vi "DetPars.vi"(1 "Immediate":bool=TRUE) -> (0 "status":i32)   [LabVIEW 2014]
uses:
  globals/DetectorGlobals.vi
panel:
  in  "FullFrame":bool caption="Boolean"
  in  "Last \nColumn":i32=4096 min=1 step=1
  in  "Last\nRow":i32=4096 min=1 step=1
  in  "Row\nBin":i32=3 min=1 max=100 step=1
  in  "Column\nBin":i32=5 min=1 max=100 step=1
  in  "First \nColumn":i32=1 min=1 step=1
  in  "First\nRow":i32=1 min=1 step=1
  in  "OK":bool caption="Boolean"
  in  "Apply":bool caption="Boolean"
  in  "Quit":bool
  in  "Close":bool caption="Boolean"
  # "Detector Region-Of-Interest"
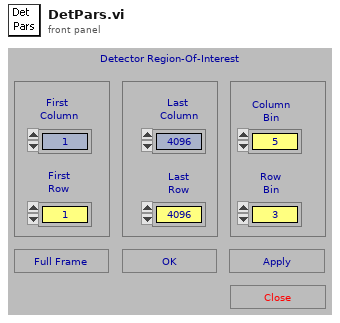
[diagram p1: front panel]
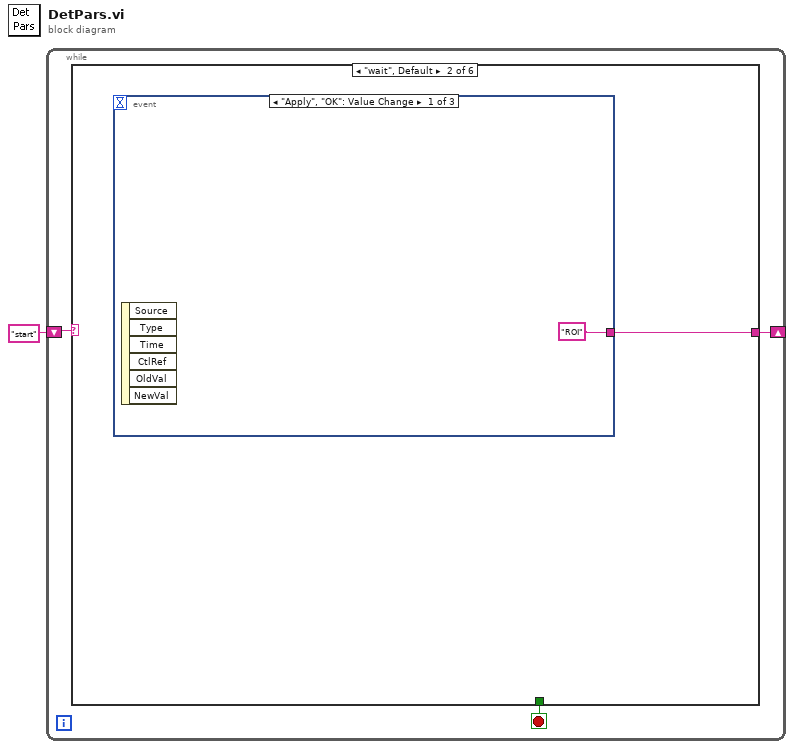
[diagram p0: block diagram]
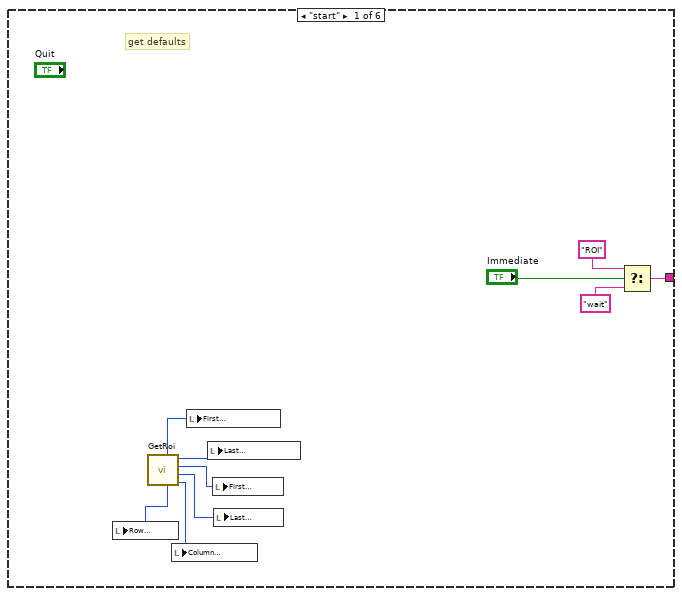
[diagram p2: hidden frame]
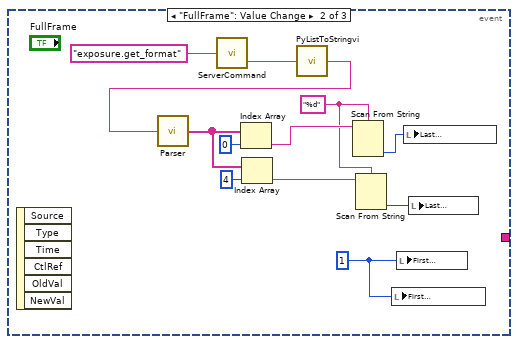
[diagram p3: hidden frame]
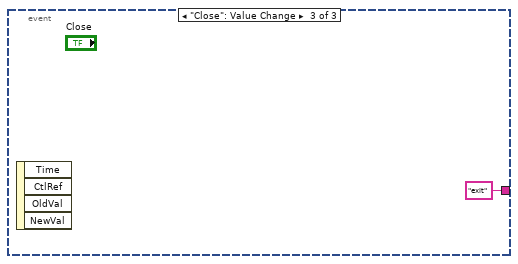
[diagram p4: hidden frame]
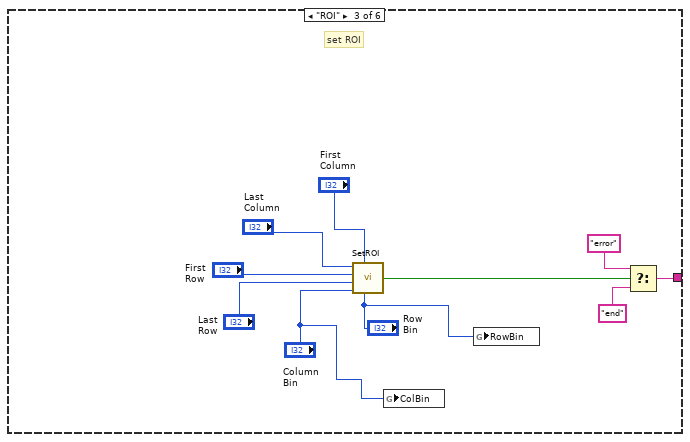
[diagram p5: hidden frame]
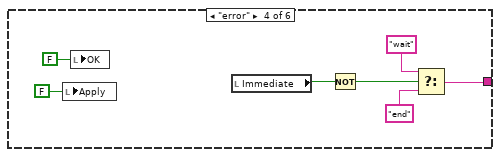
[diagram p6: hidden frame]
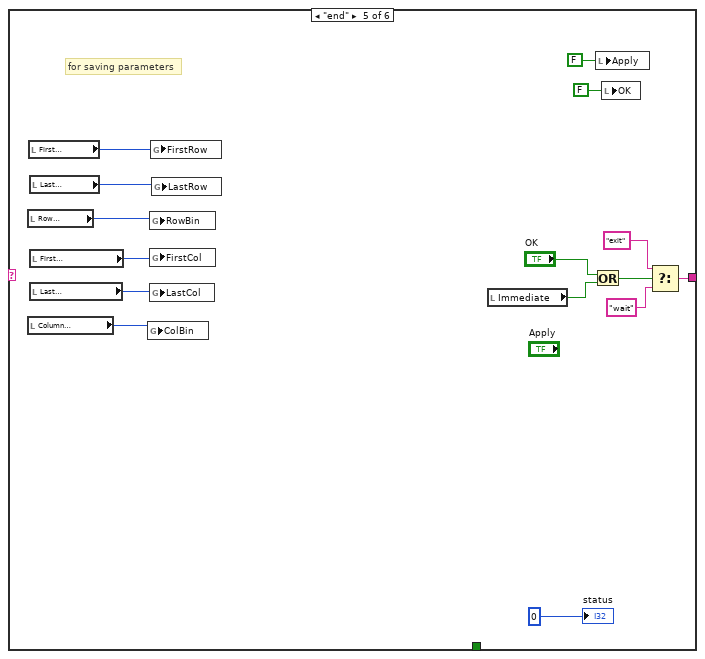
[diagram p7: hidden frame]
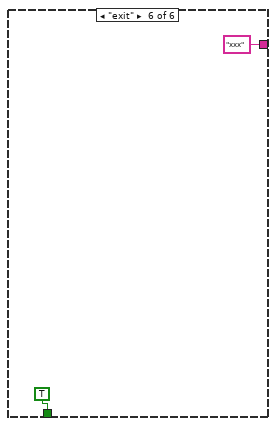
[diagram p8: hidden frame]
diagram:
  n1 = while {
    shift-right: [w3] -> _
    shift-left: "start" -> [w4]
    stop <- w2 stop-if-true
    n2 = case shown="\"wait\", Default" w4 {
      tunnel: [w14 w15 w35 w46 w60 "xxx"] -> w3
      tunnel: [_ _ _ _ _ TRUE] -> w2
      frame "start" {
        # "get defaults"
        n3 = call "GetRoi.vi"() -> ("FirstCol"=w10:i32, "RowBin"=w5:i32, "LastCol"=w9:i32, "FirstRow"=w8:i32, "LastRow"=w7:i32, "ColBin"=w6:i32)  [unwired: 1 in]
        n4 = local write "Row\nBin"(w5) -> ()
        n5 = local write "Column\nBin"(w6) -> ()
        n6 = local write "First \nColumn"(w10) -> ()
        n7 = local write "Last \nColumn"(w9) -> ()
        n8 = local write "First\nRow"(w8) -> ()
        n9 = local write "Last\nRow"(w7) -> ()
        n10 = Select(t="ROI", s="Immediate", f="wait") -> (s? t:f=w14:string)
      }
      frame "wait", Default {
        n11 = event shown="[0] \"Apply\", \"OK\": Value Change" {
          selector: _ -> [_ _ _]
          dyn-events: _ -> [_ _ _]
          timeout: _ -> [_ _ _]
          tunnel: ["ROI" _ "exit"] -> w15
          event "Apply", "OK": Value Change {
            n12 = event-data() -> ()  [unwired: 1 in, 6 out]
          }
          event "FullFrame": Value Change {
            w17 = 1 ("First\nRow")
            w18 = "%d" ("format string")
            n13 = event-data() -> ()  [unwired: 1 in, 6 out]
            n14 = call "ServerCommand.vi"("Command"="exposure.get_format") -> ("Reply"=w27:string)  [unwired: 1 out]
            n15 = call "PyListToStringvi.vi"("PythonList"=w27) -> ("String"=w26:string)
            n16 = call "Parser.vi"("string"=w26) -> ("Out Strings"=w25:string[])
            n17 = Index Array(array=w25, index=0) -> (element=w22:string)
            n18 = Index Array(array=w25, index=4) -> (element=w19:string)
            n19 = Scan From String(format string=w18, input string=w22) -> (output 1=w21:i32)  [unwired: 3 in, 3 out]
            n20 = Scan From String(format string=w18, input string=w19) -> (output 1=w20:i32)  [unwired: 3 in, 3 out]
            n21 = local write "First \nColumn"(w17) -> ()
            n22 = local write "First\nRow"(w17) -> ()
            n23 = local write "Last \nColumn"(w21) -> ()
            n24 = local write "Last\nRow"(w20) -> ()
          }
          event "Close": Value Change {
            n25 = event-data() -> ()  [unwired: 1 in, 4 out]
          }
        }
      }
      frame "ROI" {
        # "set ROI"
        n26 = call "SetROI.vi"("RowBIn"="Row\nBin", "FirstCol"="First \nColumn", "ColBin"="Column\nBin", "LastRow"="Last\nRow", "FirstRow"="First\nRow", "LastCol"="Last \nColumn") -> ("Error"=w32:bool)
        n27 = global write "DetectorGlobals.vi" "ColBin"("Column\nBin") -> ()
        n28 = global write "DetectorGlobals.vi" "RowBin"("Row\nBin") -> ()
        n29 = Select(t="error", s=w32, f="end") -> (s? t:f=w35:string)
      }
      frame "error" {
        n30 = local write "Apply"(FALSE ("Apply")) -> ()
        n31 = local write "OK"(FALSE ("OK")) -> ()
        n32 = local read "Immediate"() -> (w41:bool)
        n33 = Not(x=w41) -> (.not. x?=w40:bool)
        n34 = Select(t="wait", s=w40, f="end") -> (s? t:f=w46:string)
      }
      frame "end" {
        # "for saving parameters"
        n35 = local read "Row\nBin"() -> (w50:i32)
        n36 = local read "Column\nBin"() -> (w49:i32)
        n37 = local read "First\nRow"() -> (w52:i32)
        n38 = local read "Last\nRow"() -> (w51:i32)
        n39 = local read "First \nColumn"() -> (w47:i32)
        n40 = local read "Last \nColumn"() -> (w48:i32)
        n41 = global write "DetectorGlobals.vi" "ColBin"(w49) -> ()
        n42 = global write "DetectorGlobals.vi" "RowBin"(w50) -> ()
        n43 = global write "DetectorGlobals.vi" "FirstCol"(w47) -> ()
        n44 = global write "DetectorGlobals.vi" "LastCol"(w48) -> ()
        n45 = global write "DetectorGlobals.vi" "FirstRow"(w52) -> ()
        n46 = global write "DetectorGlobals.vi" "LastRow"(w51) -> ()
        n47 = local read "Immediate"() -> (w53:bool)
        n48 = Or(x="OK", y=w53) -> (x .or. y?=w56:bool)
        n49 = local write "Apply"(FALSE ("Apply")) -> ()
        n50 = local write "OK"(FALSE ("OK")) -> ()
        n51 = Select(t="exit", s=w56, f="wait") -> (s? t:f=w60:string)
        "status" <- 0 ("status")
      }
      frame "exit" {
      }
    }
  }
